vi "PRACH Measurement Stop.vi"(8 "error in (no error)":errorcluster, 10 "Instance (1)":T1=1, 11 "VISA resource name":refnum<visa-resource-name>) -> (0 "error out":errorcluster, 3 "VISA resource name out":refnum<visa-resource-name>)   [LabVIEW 2020, in "Rohde&Schwarz CMWXP NR FR1 Measurement.lvlib"]
doc: "Halts the measurement immediately. The measurement enters the 'OFF' state. All measurement values are set to NAV. Allocated resources are released. Use FETCh...STATe? to query the current measurement state.\n\nAttribute:\nRSCMWXPNRFR1M_ATTR_PRACH_STOP_MEASUREMENT\n\nRemote-control command:\nSTOP:NRSub:MEAS<i>:PRACh"
uses:
  <instrlib>/Rohde&Schwarz CMWXP NR FR1 Measurement/Rohde&Schwarz CMWXP NR FR1 Measurement.lvlib
  <instrlib>/Rohde&Schwarz CMWXP NR FR1 Measurement/Private/_Instance.ctl
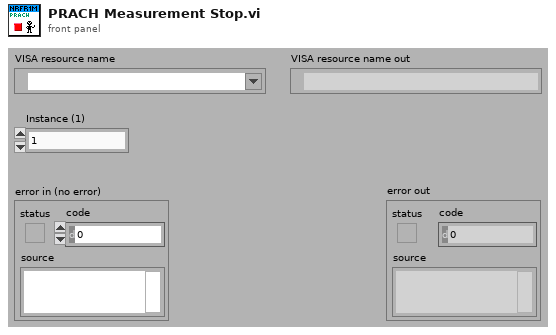
[diagram p1: front panel]
types:
  T1 = typedef "Rohde&Schwarz CMWXP NR FR1 Measurement.lvlib/_Instance.ctl" = i32
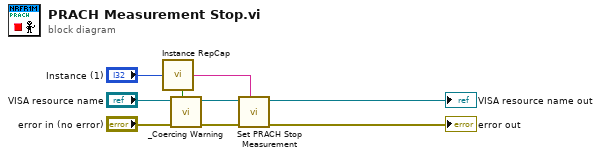
[diagram p0: block diagram]
diagram:
  n1 = call <instrlib>:"Instance RepCap.vi"("Instance In"="Instance (1)") -> ("In Range?"=w2:bool, "RepCap Identifier Out"=w1:string)  [unwired: 1 in]
  n2 = call <instrlib>:"_Coercing Warning.vi"("In Range?"=w2, "error in (no error)"="error in (no error)", "VISA resource name"="VISA resource name") -> ("error out"=w5:errorcluster, "VISA resource name out"=w4:refnum<visa-resource-name>)  [unwired: 7 in]
  n3 = call "Set PRACH Stop Measurement"("Repeated Capabilities"=w1, "error in (no error)"=w5, "instrument handle"=w4) -> ("error out"=→"error out":errorcluster, "instrument handle out"=→"VISA resource name out":refnum<visa-resource-name>)  [unwired: 7 in]
